vi "AvgByGroups2.vi"(8 "Groups2Avg":dbl, 11 "Input Graph to be Averaged":cluster{dbl[], dbl[]}(graph)) -> (3 "Output Graph after Averaging":cluster{dbl[], dbl[]}(graph))   [LabVIEW 2016]
panel:
  out "X Averaged by Groups":dbl[](array[numeric])
  out "Y Averaged by Groups":dbl[](array[numeric])
  out "size(s)":i32
  out "Y":dbl[](array[numeric])
  out "X":dbl[](array[numeric])
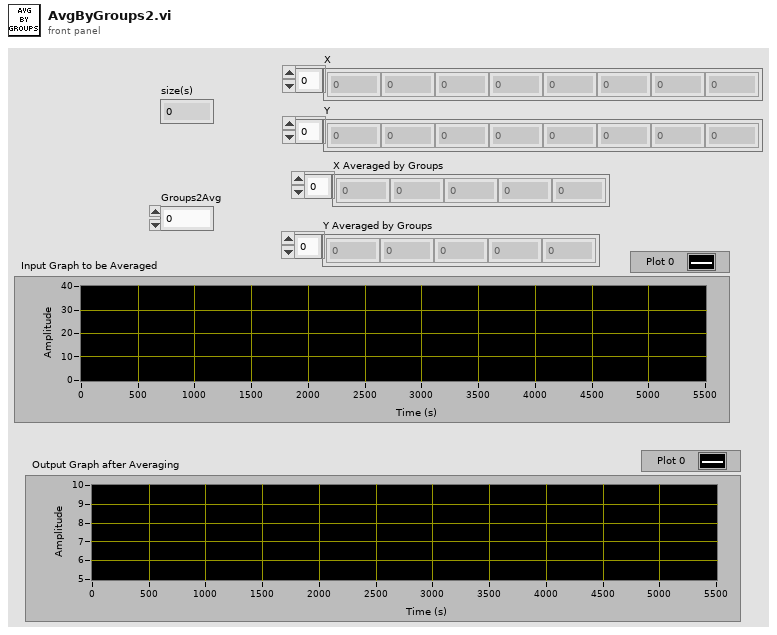
[diagram p1: front panel]
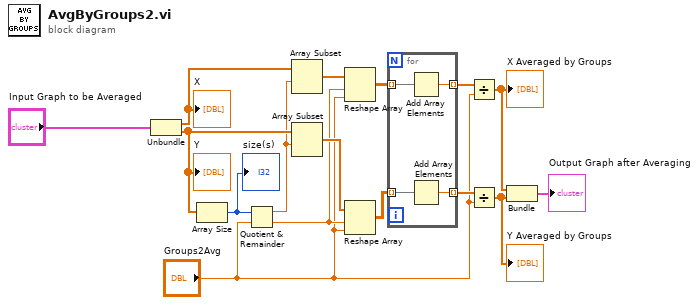
[diagram p0: block diagram]
diagram:
  n1 = Unbundle("Input Graph to be Averaged") -> (w9:dbl[], w14:dbl[])
  "X" <- w9
  "Y" <- w14
  n2 = Array Size(array=w14) -> (size(s)=w15:i32)
  "size(s)" <- w15
  n3 = Quotient & Remainder(x=w15, y="Groups2Avg") -> (x-y*floor(x/y)=w8:dbl, floor(x/y)=w7:dbl)
  n4 = Array Subset(array=w9, index=w8) -> (w10:dbl[])  [unwired: 1 in]
  n5 = Array Subset(array=w14, index=w8) -> (w13:dbl[])  [unwired: 1 in]
  n6 = Reshape Array(w10, w7, "Groups2Avg") -> (w6:dbl[][])
  n7 = Reshape Array(w13, w7, "Groups2Avg") -> (w12:dbl[][])
  n8 = for {
    tunnel: w12 -> [w20] mode=indexing
    tunnel: [w19] -> w11 mode=indexing
    tunnel: w6 -> [w18] mode=indexing
    tunnel: [w17] -> w5 mode=indexing
    n9 = Add Array Elements(numeric array=w18) -> (sum=w17:dbl)
    n10 = Add Array Elements(numeric array=w20) -> (sum=w19:dbl)
  }
  n11 = Divide(x=w5, y="Groups2Avg") -> (x/y=w3:dbl[])
  "X Averaged by Groups" <- w3
  n12 = Divide(x=w11, y="Groups2Avg") -> (x/y=w2:dbl[])
  "Y Averaged by Groups" <- w2
  n13 = Bundle(w3, w2) -> (→"Output Graph after Averaging":cluster{dbl[], dbl[]})  [unwired: 1 in]
